vi "CmdParser.vi"(11 "message":T3={"update_id"=0, "from"="", "text"="", "date"=timestamp(2082844800 s since 1904-01-01), "chat_id"=0, "type"="", "reply_to_message.text"="", "message_id"=0}) -> (0 "msg_type":string, 1 "Cmd":T2={"Cmd"=["Default", "/getweather", "/led1", "/led2", "/led3", "/gettime", "on", "off", "delete keyboard", "/start"], "Param"=[], "CmdText"="", "ChatId"=0}, 2 "chat_id":i32, 3 "message":T3={"update_id"=0, "from"="", "text"="", "date"=timestamp(2082844800 s since 1904-01-01), "chat_id"=0, "type"="", "reply_to_message.text"="", "message_id"=0})   [LabVIEW 2015]
uses:
  Telegram/Methods/TypeDefs/Message.ctl
  Telegram/Methods/TypeDefs/CommandList.ctl
panel:
  out "reply_to_message":bool
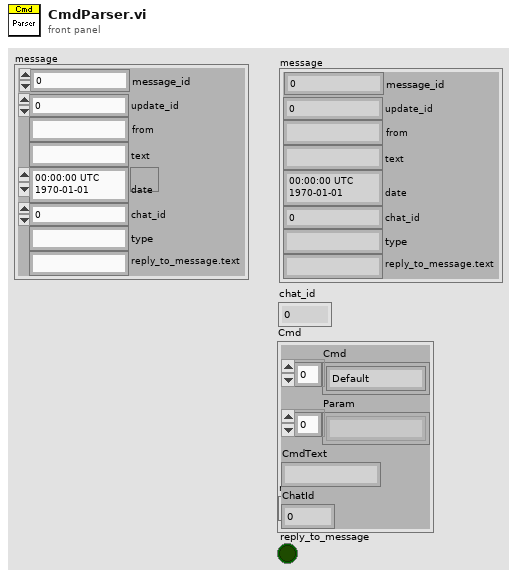
[diagram p1: front panel]
types:
  T1 = typedef "CommandList.ctl" = string[]
  T2 = cluster{"Cmd":T1, "Param":string[], "CmdText":string, "ChatId":i32}
  T3 = typedef "Message.ctl" = cluster{"update_id":u32, "from":string, "text":string, "date":timestamp, "chat_id":i32, "type":string, "reply_to_message.text":string, "message_id":u32}
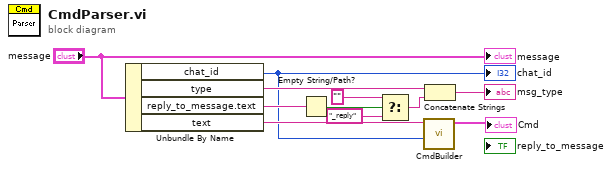
[diagram p0: block diagram]
diagram:
  n1 = Unbundle By Name("message") -> ("chat_id"=w1:i32, "type"=w4:string, "reply_to_message.text"=w5:string, "text"=w6:string)
  "chat_id" <- w1
  n2 = Empty String/Path?(string/path=w5) -> (empty?=w7:bool)
  n3 = Select(t="" ("text"), s=w7, f="_reply") -> (s? t:f=w8:string)
  n4 = call "CmdBuilder.vi"("ChatId"=w1, "InText"=w6) -> ("Cmd"=→"Cmd":T2)  [unwired: 9 in]
  n5 = Concatenate Strings(w4, w8) -> (→"msg_type":string)
  "message" <- "message"
